vi "SCB RT.vi"() -> ()   [LabVIEW 2016]
uses:
  SC2 states.ctl
  <vilib>/Platform/TimedLoop/XDataNode/timing_clust.ctl
  <vilib>/Platform/TimedLoop/XDataNode/nitl_modes.ctl
  <vilib>/Platform/TimedLoop/XDataNode/wakeup.ctl
  Encoder bit cluster.ctl
  <vilib>/Platform/TimedLoop/XDataNode/loadnilvce.vi
  <vilib>/Motion/Express/_s/nimc.fb.straightLineMove.startStraightLineMove.axis.modeRelative.0.vi
  <vilib>/Platform/TimedLoop/XDataNode/XDataNode.xnode
  <vilib>/Motion/BlockNode/FB.NIMotion.xnode
  <vilib>/Platform/TimedLoop/XDataNode/XDNodeRunTimeDep.lvlib
  <vilib>/nisyscfg/nisyscfg.lvlib
  <vilib>/nisyscfg/Find Hardware.vi
panel:
  out "Encoder displacement":i32
  in  "Random Sample":bool
  out "Within window?":bool
  in  "Stop":bool
  out "Motor status":bool=TRUE
  in  "Encoder offset":i32=-1277
  in  "Start Sample Change":bool
  out "SC2 State Control":T1=enum."wait"
  out "Encoder readback":errorcluster
  in  "error in (no error)":errorcluster
  out "status":bool
  out "Encoder destination":i32
  in  "New Move (Motor steps)":dbl=10000.0 format="%#_13g"
  in  "New Sample":i16
  in  "Step Window radius":i32=2
  out "Converted Encoder":bool[](array[boolean])
  in  "Motion Resource":refnum<k21>="Axis SCB motor"
  out "Straight Line Move":errorcluster
  out "Raw Encoder":bool[](array[boolean])
  out "Encoder rotation":u16(graph)
  out "Encoder Position":i32
  # "Encoder offset required to \n\"line up\" encoder with wheel.\nSample 64 is -1021 encoder steps\n (or +15362 steps) from the \nencoder's zero point.. Note: Sample \nand encoder numbering run in \nopposite directions"
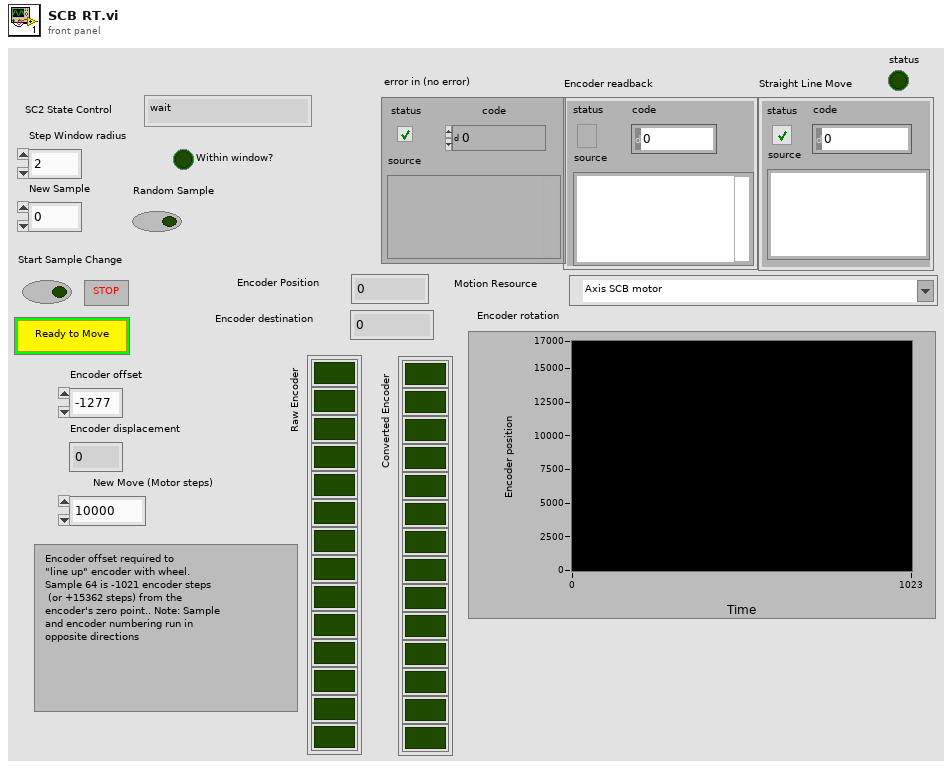
[diagram p1: front panel]
types:
  T1 = typedef "SC2 states.ctl" = enum16{"initialize", "wait", "check position", "rotate wheel", "rotate complete", "Shutdown"}
  T2 = typedef "XDNodeRunTimeDep.lvlib/timing_clust.ctl" = cluster{"Expected End [f-1]":u64, "Actual End [f-1]":u64, "Finished Late? [f-1]":bool, "Expected End [i-1]":u64, "Actual End [i-1]":u64, "Finished Late? [i-1]":bool, "Expected Start [i]":u64, "Actual Start [i]":u64, "Expected Start [f]":u64, "Actual Start [f]":u64, "Source Name":string, "Structure Name":string, "Period":i64, "Deadline":i64, "Offset":i64, "Start":i64, "Priority":i32, "Timeout":i32, "Mode":T3, "Wakeup Reason":T4, "Error":errorcluster, "Source Type":string, "Secondary Source Type":string, "Global End Time":u64, "Global Start Time":u64, "Frame Duration":u64, "Iteration Duration":u64, "Assigned CPU":i32, "I/O Scan Engine Mode":u32}
  T3 = typedef "XDNodeRunTimeDep.lvlib/nitl_modes.ctl" = enum32{"No Change", "Process missed periods, maintain original phase", "Discard missed periods, maintain original phase", "Process missed periods, ignore original phase", "Discard missed periods, ignore original phase"}
  T4 = typedef "XDNodeRunTimeDep.lvlib/wakeup.ctl" = enum32{"Normal", "Aborted", "Asynchronous wakeup", "Timing source error", "Timed loop error", "Timeout"}
  T5 = typedef "Encoder bit cluster.ctl" = cluster{"MSB":bool, "13th bit":bool, "12th bit":bool, "11th bit":bool, "10th bit":bool, "9th bit":bool, "8th bit":bool, "7th bit":bool, "6th bit":bool, "5th bit":bool, "4th bit":bool, "3rd bit":bool, "2nd bit":bool, "LSB":bool}
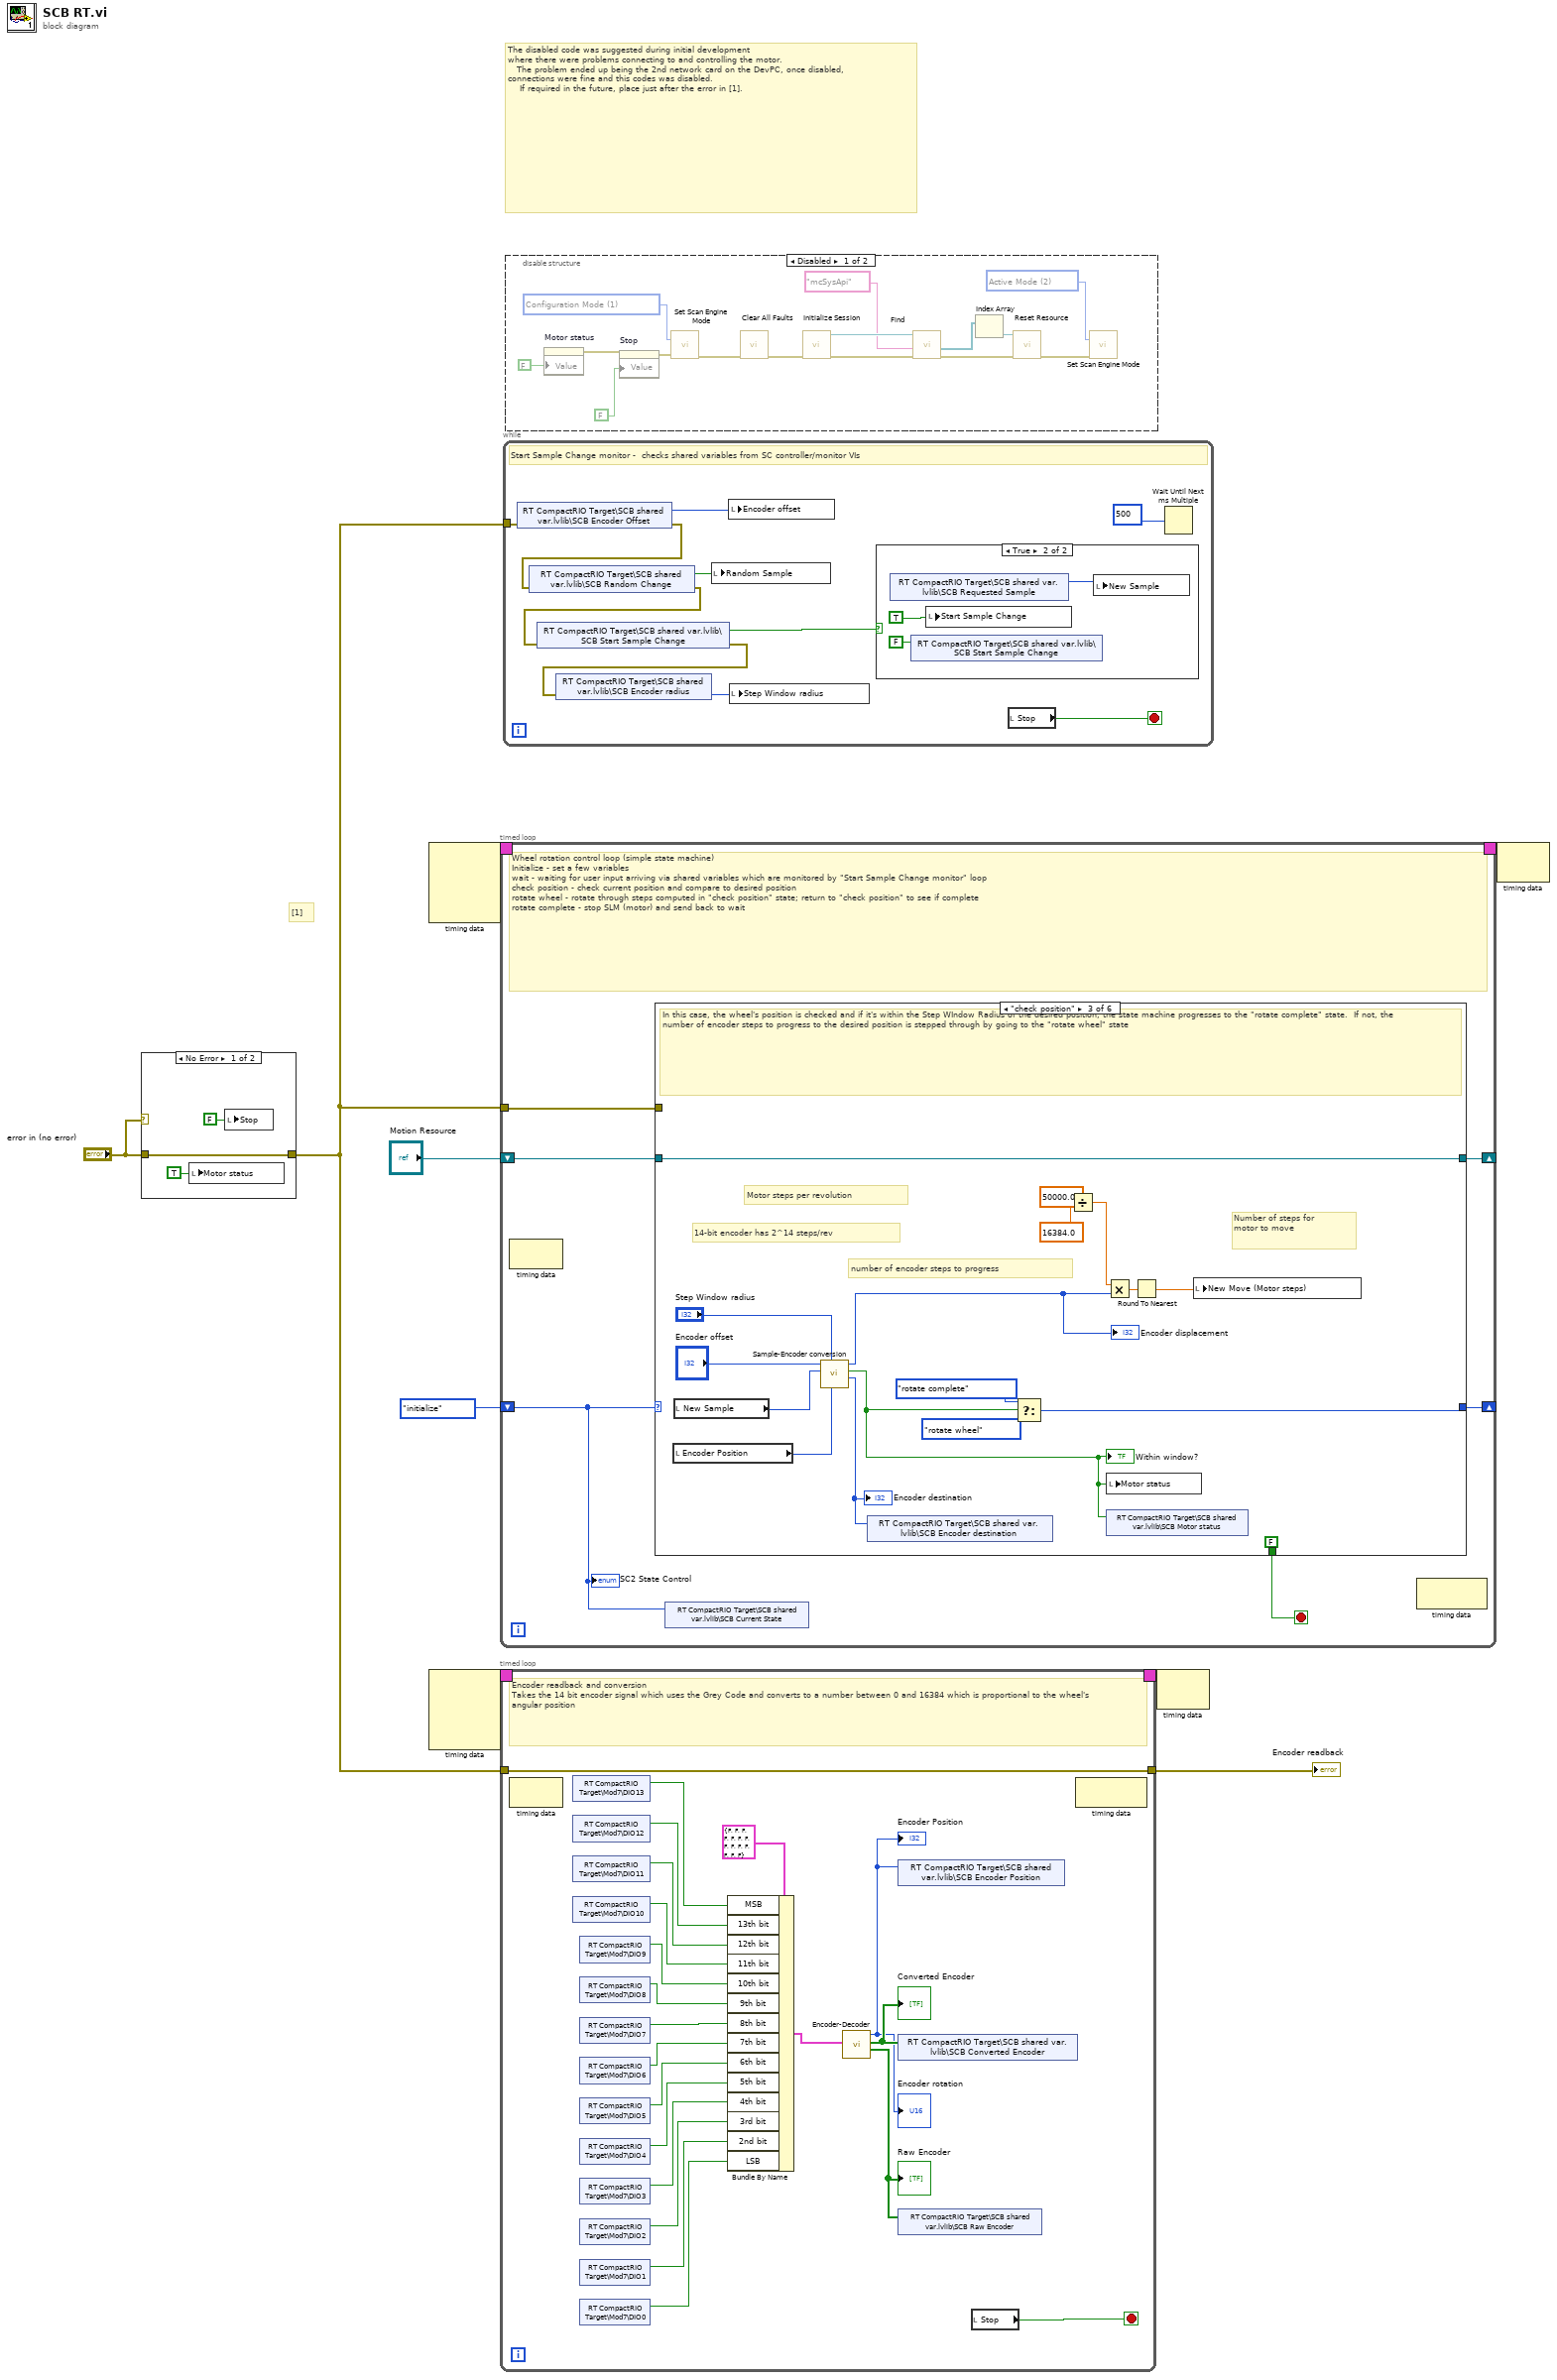
[diagram p0: block diagram]
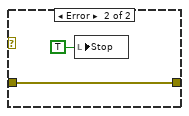
[diagram p2: hidden frame]
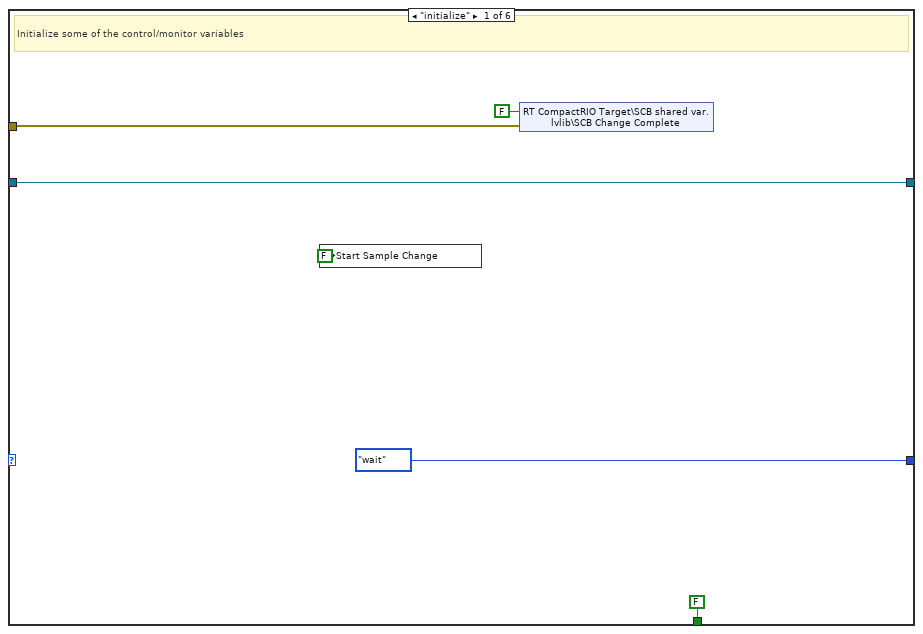
[diagram p5: hidden frame]
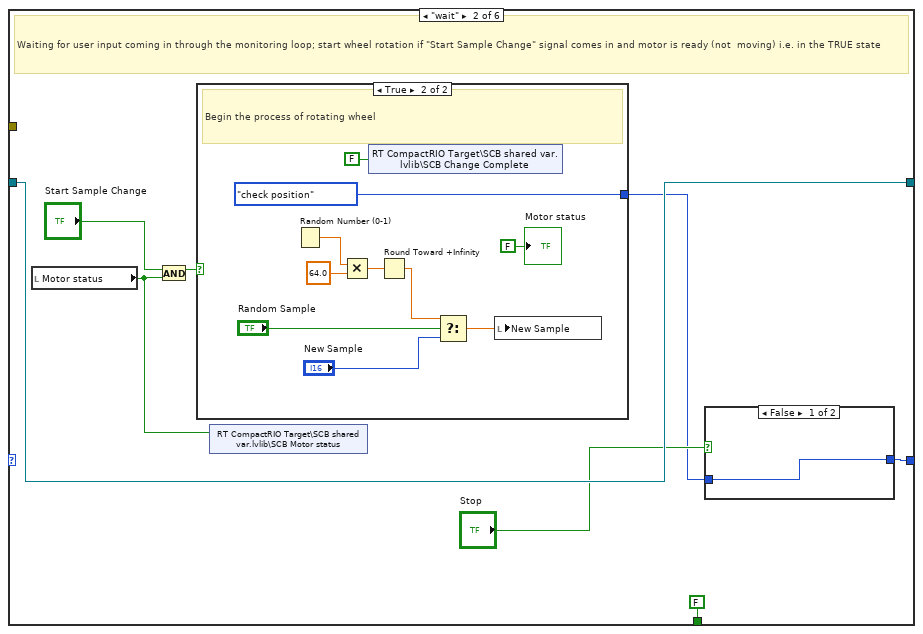
[diagram p6: hidden frame]
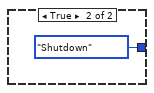
[diagram p7: hidden frame]
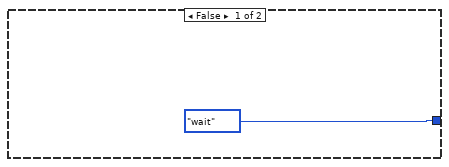
[diagram p8: hidden frame]
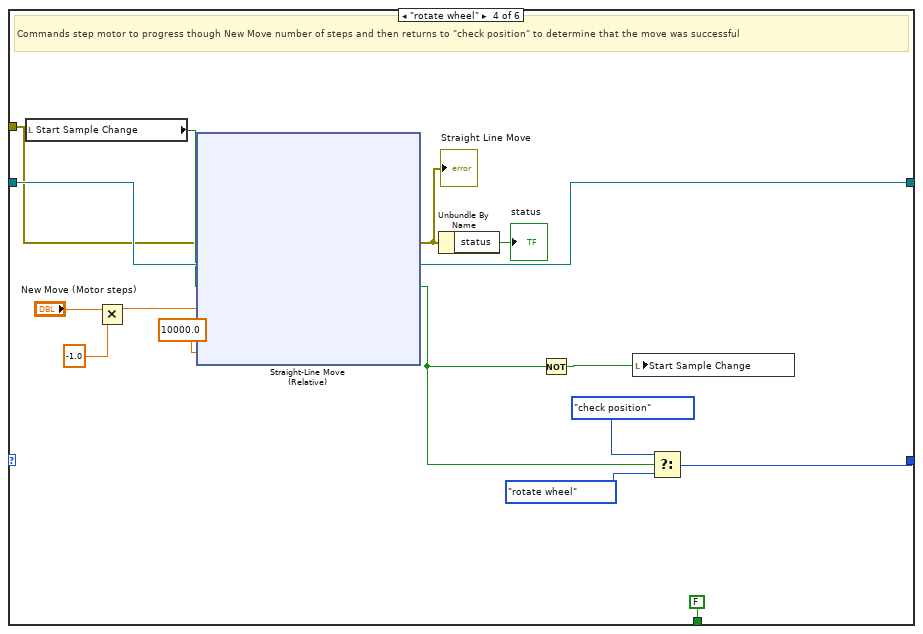
[diagram p9: hidden frame]
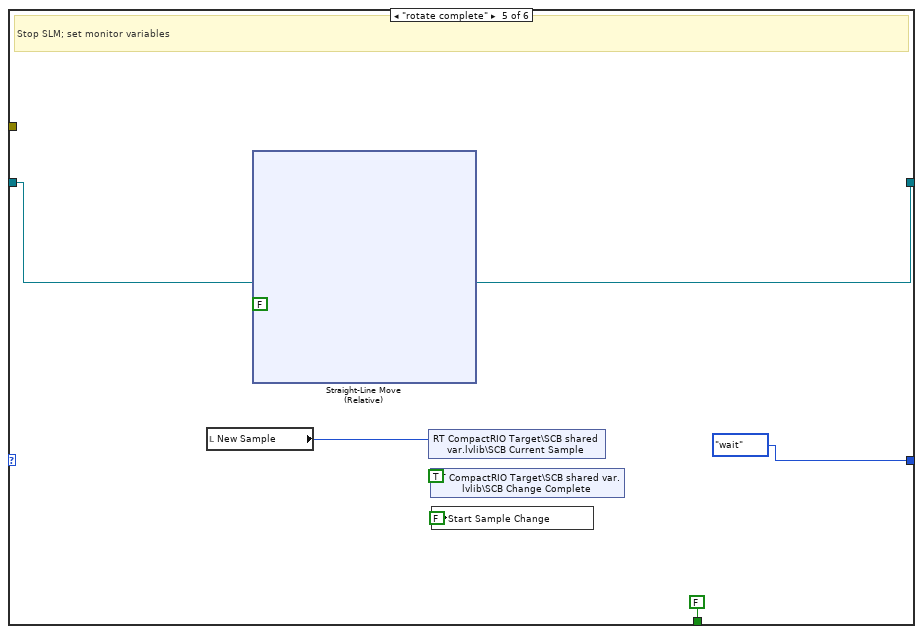
[diagram p10: hidden frame]
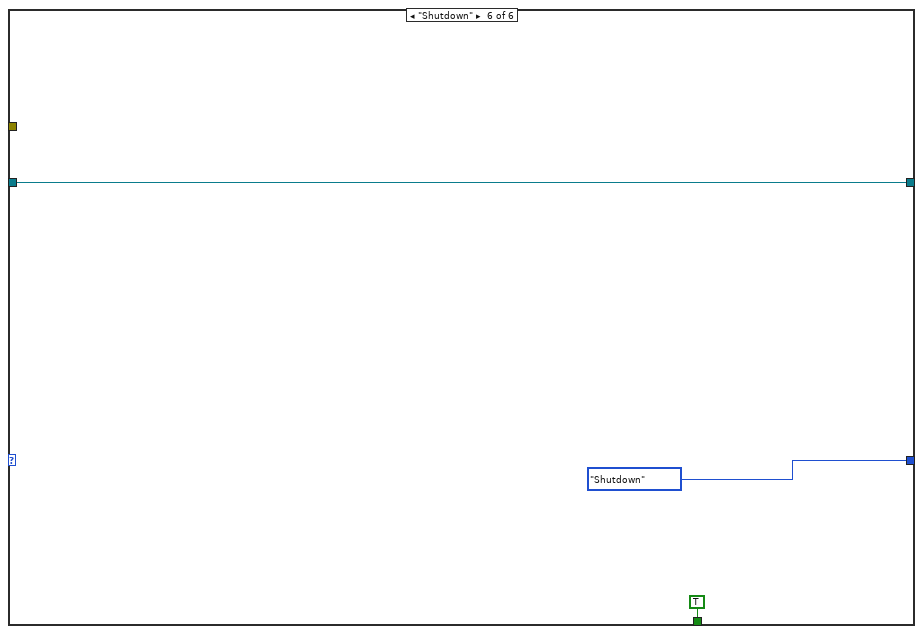
[diagram p11: hidden frame]
diagram:
  # "[1]"
  # "The disabled code was suggested during initial development\nwhere there were problems connecting to and controlling the motor.\n   The problem ended up being the 2nd network card on the DevPC, once disabled, connections were fine and this codes was disabled.  \n    If required in the future, place just after the error in [1]."
  n1 = case shown="No Error" "error in (no error)" {
    tunnel: "error in (no error)" -> [w11 w14]
    tunnel: [w11 w14] -> w2
    frame No Error {
      n2 = local write "Motor status"(TRUE ("Motor status")) -> ()
      n3 = local write "Stop"(FALSE ("Stop")) -> ()
    }
    frame Error {
      n4 = local write "Stop"(TRUE ("Stop")) -> ()
    }
  }
  n5 = node-c288() -> (w7:T2)  [unwired: 4 in]
  n6 = node-c288() -> (w9:T2)  [unwired: 4 in]
  n7 = timed-loop {
    timing: w7 -> [_]
    timing-out: [_] -> w6
    shift-right: [w19] -> _
    shift-left: SC2_states."initialize" -> [w16]
    shift-right: [w18] -> _
    shift-left: "Motion Resource" -> [w20]
    tunnel: w2 -> [w17]
    stop <- w15 stop-if-true
    # "Wheel rotation control loop (simple state machine)\nInitialize - set a few variables \nwait - waiting for user input arriving via shared variables which are monitored by \"Start Sample Change monitor\" loop\ncheck position - check current position and compare to desired position \nrotate wheel - rotate through steps computed in \"check position\" state; return to \"check position\" to see if complete\nrotate complete - stop SLM (motor) and send back to wait"
    n8 = node-c288() -> ()  [unwired: 1 in, 1 out]
    n9 = case shown="\"check position\"" w16 {
      tunnel: w20 -> [w25 w33 w51 w79 w105 w125]
      tunnel: [SC2_states."wait" w28 w64 w74 SC2_states."wait" SC2_states."Shutdown"] -> w19
      tunnel: [w25 w33 w51 w71 w102 w125] -> w18
      tunnel: w17 -> [w22 _ _ w67 _ _]
      tunnel: [FALSE FALSE FALSE FALSE FALSE TRUE] -> w15
      frame "initialize" {
        # "Initialize some of the control/monitor variables"
        n10 = local write "Start Sample Change"(FALSE ("Start Sample Change")) -> ()
        n11 = shared-variable "RT CompactRIO Target\\SCB shared var.lvlib\\SCB Change Complete"(FALSE ("SC2 Change Complete"), error in=w22) -> ()  [unwired: 1 out]
      }
      frame "wait" {
        # "Waiting for user input coming in through the monitoring loop; start wheel rotation if \"Start Sample Change\" signal comes in and motor is ready (not  moving) i.e. in the TRUE state"
        n12 = local read "Motor status"() -> (w31:bool)
        n13 = And(x="Start Sample Change", y=w31) -> (x .and. y?=w32:bool)
        n14 = case shown="True" w32 {
          tunnel: [SC2_states."wait" SC2_states."check position"] -> w29
          frame False {
          }
          frame True {
            # "Begin the process of rotating wheel"
            n15 = Random Number (0-1)() -> (number: 0 to 1=w46:dbl)
            n16 = Multiply(x=w46, y=64.0) -> (x*y=w47:dbl)
            n17 = shared-variable "RT CompactRIO Target\\SCB shared var.lvlib\\SCB Change Complete"(FALSE) -> ()  [unwired: 1 in, 1 out]
            n18 = Round Toward +Infinity(x=w47) -> (ceil(x): smallest int >= x=w41:dbl)
            n19 = Select(t=w41, s="Random Sample", f="New Sample") -> (s? t:f=w40:dbl)
            n20 = local write "New Sample"(w40) -> ()
            "Motor status" <- FALSE ("Motor status")
          }
        }
        n21 = shared-variable "RT CompactRIO Target\\SCB shared var.lvlib\\SCB Motor status"(w31) -> ()  [unwired: 1 in, 1 out]
        n22 = case shown="False" "Stop" {
          tunnel: [w35 SC2_states."Shutdown"] -> w28
          tunnel: w29 -> [w35 _]
          frame False {
          }
          frame True {
          }
        }
      }
      frame "check position" {
        # "Number of steps for\nmotor to move"
        # "number of encoder steps to progress"
        # "14-bit encoder has 2^14 steps/rev"
        # "Motor steps per revolution"
        # "In this case, the wheel's position is checked and if it's within the Step WIndow Radius of the desired position, the state machine progresses to the \"rotate complete\" state.  If not, the number of encoder steps to progress to the desired position is stepped through by going to the \"rotate wheel\" state"
        n23 = local read "Encoder Position"() -> (w58:i32)
        n24 = local read "New Sample"() -> (w50:i16)
        n25 = call "Sample-Encoder conversion.vi"("Encoder Position"=w58, "Step Window radius"="Step Window radius", "New Sample Number"=w50, "Encoder offset"="Encoder offset") -> ("Encoder destination"=w56:i32, "Within Range?"=w49:bool, "Encoder displacement"=w59:i32)  [unwired: 5 in]
        "Encoder destination" <- w56
        "Within window?" <- w49
        "Encoder displacement" <- w59
        n26 = shared-variable "RT CompactRIO Target\\SCB shared var.lvlib\\SCB Encoder destination"(w56) -> ()  [unwired: 1 in, 1 out]
        n27 = Select(t=SC2_states."rotate complete", s=w49, f=SC2_states."rotate wheel") -> (s? t:f=w64:T1)
        n28 = Divide(x=50000.0, y=16384.0) -> (x/y=w63:dbl)
        n29 = Multiply(x=w63, y=w59) -> (x*y=w60:dbl)
        n30 = local write "Motor status"(w49) -> ()
        n31 = shared-variable "RT CompactRIO Target\\SCB shared var.lvlib\\SCB Motor status"(w49) -> ()  [unwired: 1 in, 1 out]
        n32 = Round To Nearest(number=w60) -> (nearest integer value=w53:dbl)
        n33 = local write "New Move (Motor steps)"(w53) -> ()
      }
      frame "rotate wheel" {
        w80 = 10000.0
        # "Commands step motor to progress though New Move number of steps and then returns to \"check position\" to determine that the move was successful"
        n34 = local read "Start Sample Change"() -> (w75:bool)
        n35 = Multiply(x="New Move (Motor steps)", y=-1.0) -> (x*y=w70:dbl)
        n36 = xnode "Straight-Line Move\n(Relative)"("error in"=w67, "resource"=w79, "execute"=w75, "position"=w70, "velocity"=w80, "acceleration"=w80) -> ("error out"=w68:errorcluster, "resource out"=w71:refnum<k21>, "done"=w72:bool)
        "Straight Line Move" <- w68
        n37 = Unbundle By Name(w68) -> ("status"=→"status":bool)
        n38 = Not(x=w72) -> (.not. x?=w66:bool)
        n39 = local write "Start Sample Change"(w66) -> ()
        n40 = Select(t=SC2_states."check position", s=w72, f=SC2_states."rotate wheel") -> (s? t:f=w74:T1)
      }
      frame "rotate complete" {
        # "Stop SLM; set monitor variables"
        n41 = local read "New Sample"() -> (w100:i16)
        n42 = xnode "Straight-Line Move\n(Relative)"("resource"=w105, "execute"=FALSE) -> ("resource out"=w102:refnum<k21>)  [unwired: 4 in, 2 out]
        n43 = shared-variable "RT CompactRIO Target\\SCB shared var.lvlib\\SCB Current Sample"(w100) -> ()  [unwired: 1 in, 1 out]
        n44 = shared-variable "RT CompactRIO Target\\SCB shared var.lvlib\\SCB Change Complete"(TRUE ("SC2 Change Complete")) -> ()  [unwired: 1 in, 1 out]
        n45 = local write "Start Sample Change"(FALSE ("Start Sample Change")) -> ()
      }
      frame "Shutdown" {
      }
    }
    n46 = shared-variable "RT CompactRIO Target\\SCB shared var.lvlib\\SCB Current State"(w16) -> ()  [unwired: 1 in, 1 out]
    n47 = node-c288() -> ()  [unwired: 1 in, 1 out]
    "SC2 State Control" <- w16
  }
  n48 = timed-loop {
    timing: w9 -> [_]
    timing-out: [_] -> w8
    tunnel: w2 -> [w145]
    tunnel: [w145] -> w3
    stop <- w128 stop-if-true
    # "Encoder readback and conversion\nTakes the 14 bit encoder signal which uses the Grey Code and converts to a number between 0 and 16384 which is proportional to the wheel's angular position"
    n49 = node-c288() -> ()  [unwired: 1 in, 1 out]
    n50 = shared-variable "RT CompactRIO Target\\Mod7\\DIO13"() -> (w144:bool)  [unwired: 1 in, 1 out]
    n51 = shared-variable "RT CompactRIO Target\\Mod7\\DIO12"() -> (w143:bool)  [unwired: 1 in, 1 out]
    n52 = shared-variable "RT CompactRIO Target\\Mod7\\DIO11"() -> (w142:bool)  [unwired: 1 in, 1 out]
    n53 = shared-variable "RT CompactRIO Target\\Mod7\\DIO10"() -> (w141:bool)  [unwired: 1 in, 1 out]
    n54 = shared-variable "RT CompactRIO Target\\Mod7\\DIO9"() -> (w140:bool)  [unwired: 1 in, 1 out]
    n55 = shared-variable "RT CompactRIO Target\\Mod7\\DIO8"() -> (w139:bool)  [unwired: 1 in, 1 out]
    n56 = shared-variable "RT CompactRIO Target\\Mod7\\DIO7"() -> (w138:bool)  [unwired: 1 in, 1 out]
    n57 = shared-variable "RT CompactRIO Target\\Mod7\\DIO6"() -> (w137:bool)  [unwired: 1 in, 1 out]
    n58 = shared-variable "RT CompactRIO Target\\Mod7\\DIO5"() -> (w136:bool)  [unwired: 1 in, 1 out]
    n59 = shared-variable "RT CompactRIO Target\\Mod7\\DIO4"() -> (w135:bool)  [unwired: 1 in, 1 out]
    n60 = shared-variable "RT CompactRIO Target\\Mod7\\DIO3"() -> (w134:bool)  [unwired: 1 in, 1 out]
    n61 = shared-variable "RT CompactRIO Target\\Mod7\\DIO2"() -> (w133:bool)  [unwired: 1 in, 1 out]
    n62 = shared-variable "RT CompactRIO Target\\Mod7\\DIO1"() -> (w132:bool)  [unwired: 1 in, 1 out]
    n63 = shared-variable "RT CompactRIO Target\\Mod7\\DIO0"() -> (w131:bool)  [unwired: 1 in, 1 out]
    n64 = Bundle By Name(cluster=T5 {"MSB"=FALSE, "13th bit"=FALSE, "12th bit"=FALSE, "11th bit"=FALSE, "10th bit"=FALSE, "9th bit"=FALSE, "8th bit"=FALSE, "7th bit"=FALSE, "6th bit"=FALSE, "5th bit"=FALSE, "4th bit"=FALSE, "3rd bit"=FALSE, "2nd bit"=FALSE, "LSB"=FALSE} ("Cluster"), "MSB"=w144, "13th bit"=w143, "12th bit"=w142, "11th bit"=w141, "10th bit"=w140, "9th bit"=w139, "8th bit"=w138, "7th bit"=w137, "6th bit"=w136, "5th bit"=w135, "4th bit"=w134, "3rd bit"=w133, "2nd bit"=w132, "LSB"=w131) -> (w129:T5)
    n65 = call "Encoder-Decoder.vi"("Encoder data"=w129) -> ("Raw bits"=w146:bool[], "Converted bits"=w148:bool[], "Encoder position"=w147:u16)  [unwired: 8 in]
    "Encoder Position" <- w147
    "Encoder rotation" <- w147
    "Raw Encoder" <- w146
    "Converted Encoder" <- w148
    n66 = shared-variable "RT CompactRIO Target\\SCB shared var.lvlib\\SCB Encoder Position"(w147) -> ()  [unwired: 1 in, 1 out]
    n67 = shared-variable "RT CompactRIO Target\\SCB shared var.lvlib\\SCB Converted Encoder"(w148) -> ()  [unwired: 1 in, 1 out]
    n68 = shared-variable "RT CompactRIO Target\\SCB shared var.lvlib\\SCB Raw Encoder"(w146) -> ()  [unwired: 1 in, 1 out]
    n69 = local read "Stop"() -> (w128:bool)
    n70 = node-c288() -> ()  [unwired: 1 in, 1 out]
  }
  "Encoder readback" <- w3
  n71 = while {
    tunnel: w2 -> [w152]
    stop <- w151 stop-if-true
    # "Start Sample Change monitor -  checks shared variables from SC controller/monitor VIs"
    n72 = shared-variable "RT CompactRIO Target\\SCB shared var.lvlib\\SCB Encoder Offset"(error in=w152) -> (w158:i16, error out=w157:errorcluster)
    n73 = shared-variable "RT CompactRIO Target\\SCB shared var.lvlib\\SCB Random Change"(error in=w157) -> (w155:bool, error out=w156:errorcluster)
    n74 = shared-variable "RT CompactRIO Target\\SCB shared var.lvlib\\SCB Start Sample Change"(error in=w156) -> (w160:bool, error out=w153:errorcluster)
    n75 = shared-variable "RT CompactRIO Target\\SCB shared var.lvlib\\SCB Encoder radius"(error in=w153) -> (w154:i32)  [unwired: 1 out]
    n76 = local write "Random Sample"(w155) -> ()
    n77 = local write "Encoder offset"(w158) -> ()
    n78 = local write "Step Window radius"(w154) -> ()
    n79 = case shown="True" w160 {
      frame False {
      }
      frame True {
        n80 = shared-variable "RT CompactRIO Target\\SCB shared var.lvlib\\SCB Requested Sample"() -> (w162:u8)  [unwired: 1 in, 1 out]
        n81 = shared-variable "RT CompactRIO Target\\SCB shared var.lvlib\\SCB Start Sample Change"(FALSE ("Start Sample Change")) -> ()  [unwired: 1 in, 1 out]
        n82 = local write "Start Sample Change"(TRUE ("Start Sample Change")) -> ()
        n83 = local write "New Sample"(w162) -> ()
      }
    }
    n84 = local read "Stop"() -> (w151:bool)
    n85 = Wait Until Next ms Multiple(millisecond multiple=500) -> ()  [unwired: 1 out]
  }
  n86 = disable-structure shown="Disabled" {
    frame Disabled {
      w170 = 2 items=["Configuration Mode"=1, "Active Mode"=2] ("mode (Active Mode)")
      w172 = 1 items=["Configuration Mode"=1, "Active Mode"=2] ("mode (Active Mode)")
      n87 = property on="Motor status" class="Bool (strict)"("Value"=FALSE ("Motor status")) -> (error out=w164:errorcluster)  [unwired: 2 in, 1 out]
      n88 = property on="Stop" class="Bool (strict)"(error in=w164, "Value"=FALSE ("Stop")) -> (error out=w166:errorcluster)  [unwired: 1 in, 1 out]
      n89 = call <vilib>:"Set Scan Engine Mode.vi"("mode (Active Mode)"=w172, "error in (no error)"=w166) -> ("error out"=w169:errorcluster)  [unwired: 13 in]
      n90 = call <vilib>:"Clear All Faults.vi"("error in (no error)"=w169) -> ("error out"=w176:errorcluster)  [unwired: 10 in]
      n91 = call <vilib>:"Initialize Session.vi"("error in (no error)"=w176) -> ("error out"=w177:errorcluster, "Session out"=w178:refnum<k21>)  [unwired: 9 in]
      n92 = call-poly <vilib>:"Find.vi"("error in (no error)"=w177, "Experts"="mcSysApi" ("experts"), "Session in"=w178) -> ("error out"=w168:errorcluster, "Resources out"=w174:refnum<k20>[])  [unwired: 5 in, 2 out]
      n93 = Index Array(array=w174) -> (element=w175:refnum<k20>)  [unwired: 1 in]
      n94 = call <vilib>:"Reset Resource.vi"("error in (no error)"=w168, "Resource in"=w175) -> ("error out"=w171:errorcluster)  [unwired: 6 in, 3 out]
      n95 = call <vilib>:"Set Scan Engine Mode.vi"("mode (Active Mode)"=w170, "error in (no error)"=w171) -> ()  [unwired: 13 in, 1 out]
    }
    frame Enabled {
    }
  }
  n96 = node-c288(w8) -> ()  [unwired: 1 out]
  n97 = node-c288(w6) -> ()  [unwired: 1 out]
